vi "Default Instrument Setup.vi"(0 "VISA resource name":refnum<visa-resource-name>, 5 "error in (no error)":errorcluster) -> (14 "VISA resource name out":refnum<visa-resource-name>, 19 "error out":errorcluster)   [LabVIEW 2020, in "Keithley 2000.lvlib"]
doc: "This Utility VI sends a default command string to the instrument whenever a new VISA session is opened, or the instrument is reset. This VI is intended to be used as a subVI for the Initialize and Reset VI's. Altering this VI could cause these two VI's to operate incorrectly."
uses:
  <instrlib>/Keithley 2000/Keithley 2000.lvlib
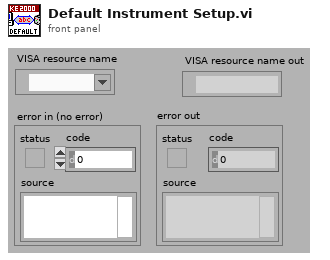
[diagram p1: front panel]
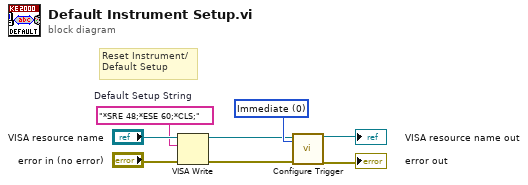
[diagram p0: block diagram]
diagram:
  w5 = u16 0 items=["Immediate", "Timer", "Manual", "Bus", "External"] ("Source (0: Immediate)")
  w6 = "*SRE 48;*ESE 60;*CLS;"  # Default Setup String
  # "Reset Instrument/\nDefault Setup"
  n1 = VISA Write(VISA resource name="VISA resource name", write buffer=w6, error in (no error)="error in (no error)") -> (VISA resource name out=w4:refnum<visa-resource-name>, error out=w3:errorcluster)  [unwired: 1 out]
  n2 = call <instrlib>:"Configure Trigger.vi"("VISA resource name"=w4, "Source (0: Immediate)"=w5, "error in (no error)"=w3) -> ("VISA resource name out"=→"VISA resource name out":refnum<visa-resource-name>, "error out"=→"error out":errorcluster)  [unwired: 15 in]
